vi "buildingDataToUpdate.vi"(11 "dataReadingToUpdate":T1) -> (2 "RawIndexToModifyOut":i32[](array[numeric]), 3 "ItemNamesOut":string[][](array[string]))   [LabVIEW 2014]
panel:
  out "dataReadingIn":T1
  in  "ItemNames":string[][](array[string])
  in  "RawIndexToModify":i32[](array[numeric])
  # "Datos a modificar en la logica del VI"
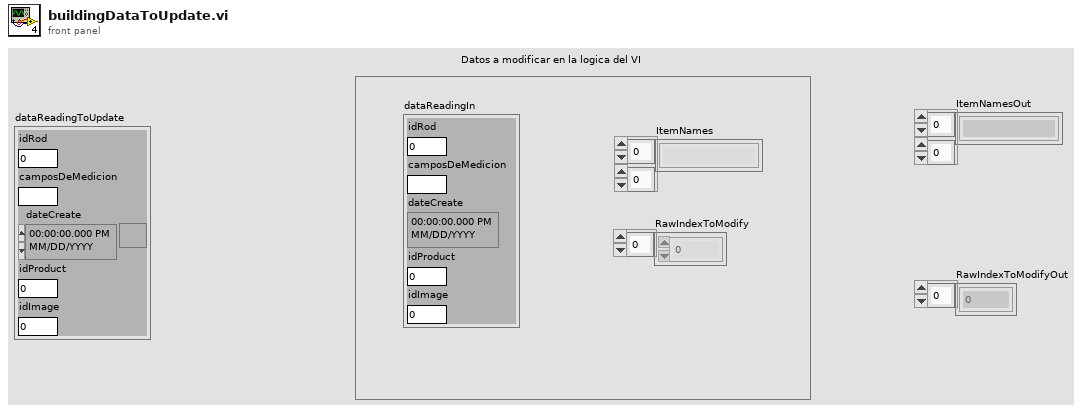
[diagram p1: front panel]
types:
  T1 = cluster{"idRod":dbl, "camposDeMedicion":string, "dateCreate":timestamp, "idProduct":dbl, "idImage":dbl}
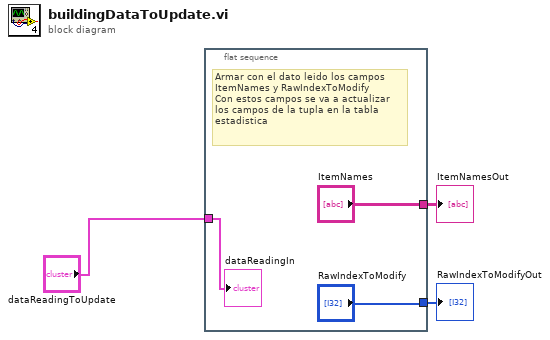
[diagram p0: block diagram]
diagram:
  n1 = flat-sequence {
    tunnel: ["RawIndexToModify"] -> w2
    tunnel: ["ItemNames"] -> w3
    tunnel: "dataReadingToUpdate" -> [w4]
    frame #0 {
      # "Armar con el dato leido los campos \nItemNames y RawIndexToModify\nCon estos campos se va a actualizar \nlos campos de la tupla en la tabla\nestadistica"
      "dataReadingIn" <- w4
    }
  }
  "ItemNamesOut" <- w3
  "RawIndexToModifyOut" <- w2
